vi "Nav Testing 2.0.vi"(11 "Start X":dbl) -> ()   [LabVIEW 2015]
panel:
  in  "String":string
  out "Array 5":dbl[][](array[numeric])
  out "x+y 2":dbl
  out "cornerDist1":dbl
  in  "Dest Y":dbl
  in  "Dest X":dbl
  in  "Start Y":dbl
  # "Moves robot between two specified points.\nNo localization data required.\n\nImplements basic motor control."
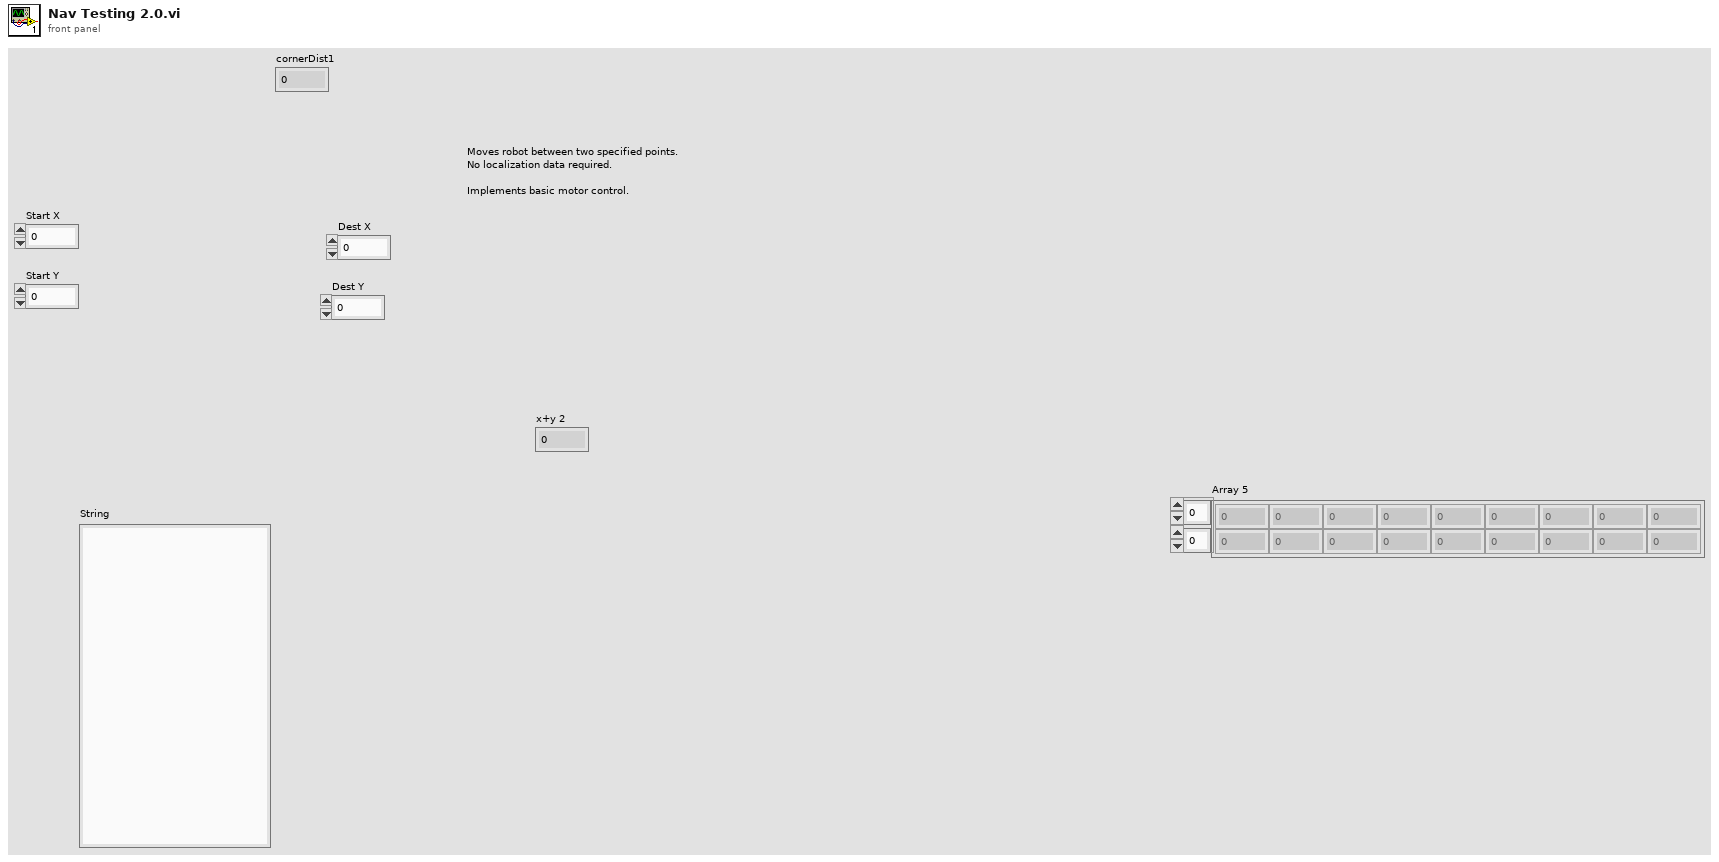
[diagram p1: front panel]
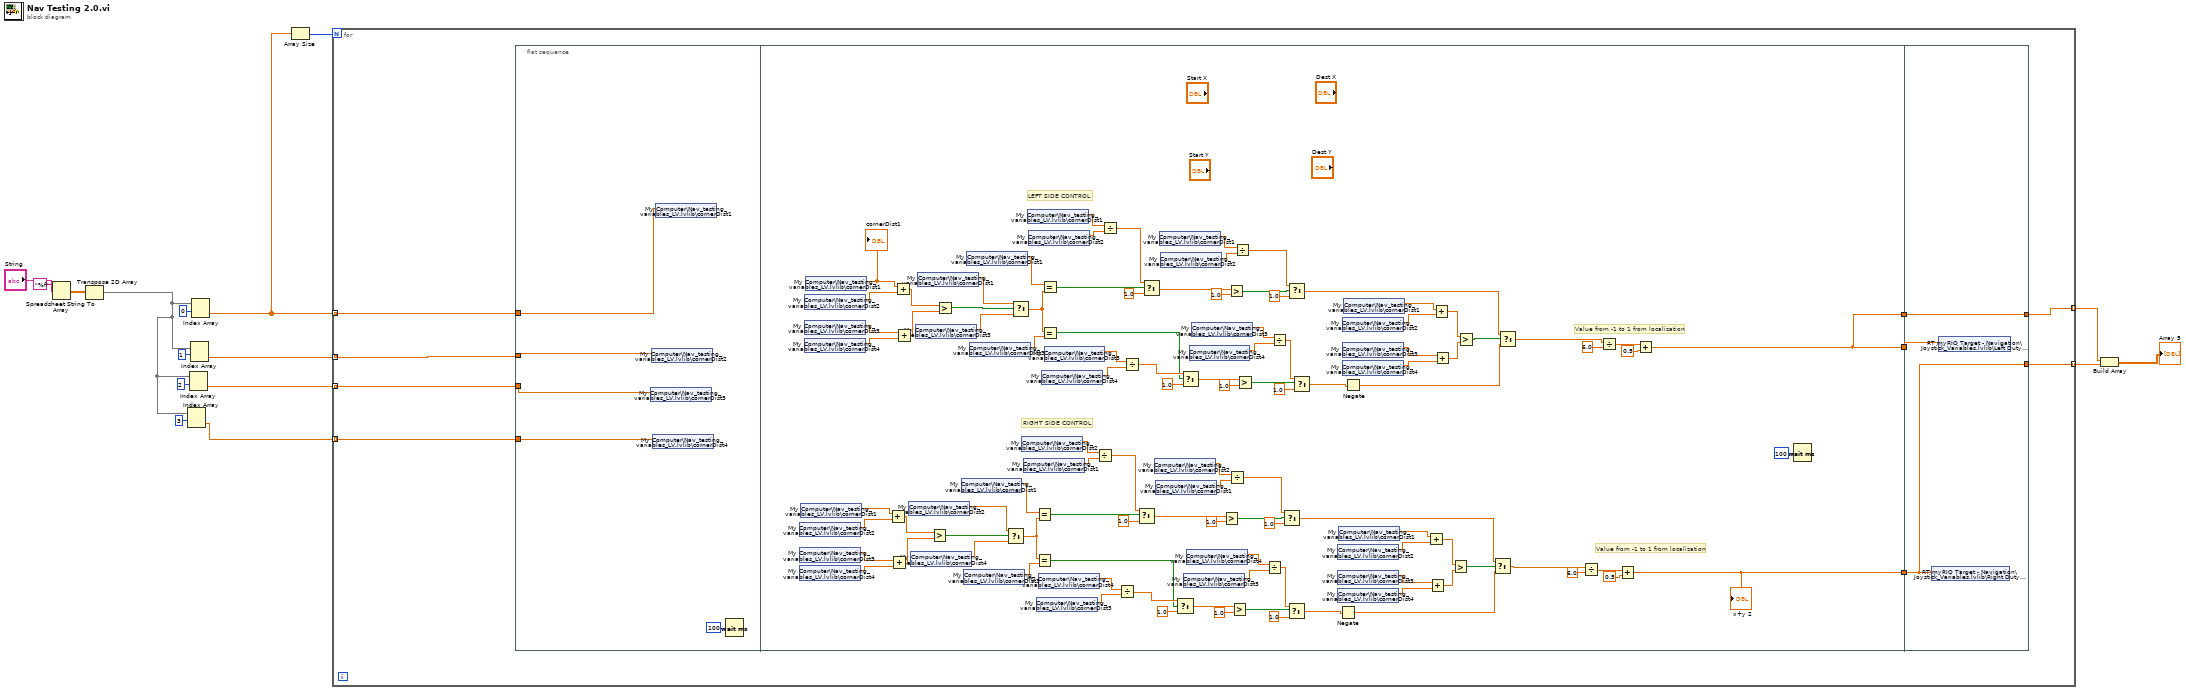
[diagram p0: block diagram]
diagram:
  n1 = Spreadsheet String To Array(format string="%f", spreadsheet string="String") -> (array=w3:dbl[][])  [unwired: 2 in]
  n2 = Transpose 2D Array(2D array=w3) -> (transposed array=w2:dbl[][])
  n3 = Index Array(array=w2, index (row)=3) -> (element=w6:dbl[])  [unwired: 1 in]
  n4 = Index Array(array=w2, index (row)=2) -> (element=w8:dbl[])  [unwired: 1 in]
  n5 = Index Array(array=w2, index (row)=1) -> (element=w10:dbl[])  [unwired: 1 in]
  n6 = Index Array(array=w2, index (row)=0) -> (element=w5:dbl[])  [unwired: 1 in]
  n7 = Array Size(array=w5) -> (size(s)=w16:i32)
  n8 = for {
    N: w16 -> [_]
    tunnel: [w22] -> w15 mode=indexing
    tunnel: w5 -> [w21] mode=indexing
    tunnel: w10 -> [w20] mode=indexing
    tunnel: w8 -> [w19] mode=indexing
    tunnel: w6 -> [w18] mode=indexing
    tunnel: [w17] -> w1 mode=indexing
    n9 = flat-sequence {
      tunnel: w21 -> [w29]
      tunnel: w20 -> [w28]
      tunnel: w19 -> [w27]
      tunnel: w18 -> [w26]
      tunnel: [w31] -> w25
      tunnel: [w32] -> w24
      tunnel: [w31] -> w23
      tunnel: w25 -> [w135]
      tunnel: w24 -> [w134]
      tunnel: w23 -> [w136]
      tunnel: [w136] -> w22
      tunnel: [w134] -> w17
      frame #0 {
        n10 = shared-variable "My Computer\\Nav_testing_variables_LV.lvlib\\cornerDist3"(w27) -> ()  [unwired: 1 in, 1 out]
        n11 = shared-variable "My Computer\\Nav_testing_variables_LV.lvlib\\cornerDist2"(w28) -> ()  [unwired: 1 in, 1 out]
        n12 = shared-variable "My Computer\\Nav_testing_variables_LV.lvlib\\cornerDist4"(w26) -> ()  [unwired: 1 in, 1 out]
        n13 = shared-variable "My Computer\\Nav_testing_variables_LV.lvlib\\cornerDist1"(w29) -> ()  [unwired: 1 in, 1 out]
        n14 = Wait (ms)(milliseconds to wait=u32 100) -> ()  [unwired: 1 out]
      }
      frame #1 {
        # "RIGHT SIDE CONTROL"
        # "LEFT SIDE CONTROL"
        # "Value from -1 to 1 from localization"
        # "Value from -1 to 1 from localization"
        n15 = shared-variable "My Computer\\Nav_testing_variables_LV.lvlib\\cornerDist2"() -> (w76:dbl)  [unwired: 1 in, 1 out]
        n16 = shared-variable "My Computer\\Nav_testing_variables_LV.lvlib\\cornerDist3"() -> (w79:dbl)  [unwired: 1 in, 1 out]
        n17 = shared-variable "My Computer\\Nav_testing_variables_LV.lvlib\\cornerDist4"() -> (w78:dbl)  [unwired: 1 in, 1 out]
        n18 = shared-variable "My Computer\\Nav_testing_variables_LV.lvlib\\cornerDist1"() -> (w77:dbl)  [unwired: 1 in, 1 out]
        n19 = shared-variable "My Computer\\Nav_testing_variables_LV.lvlib\\cornerDist2"() -> (w121:dbl)  [unwired: 1 in, 1 out]
        n20 = shared-variable "My Computer\\Nav_testing_variables_LV.lvlib\\cornerDist3"() -> (w124:dbl)  [unwired: 1 in, 1 out]
        n21 = shared-variable "My Computer\\Nav_testing_variables_LV.lvlib\\cornerDist4"() -> (w123:dbl)  [unwired: 1 in, 1 out]
        n22 = shared-variable "My Computer\\Nav_testing_variables_LV.lvlib\\cornerDist1"() -> (w122:dbl)  [unwired: 1 in, 1 out]
        "cornerDist1" <- w122
        n23 = Add(x=w77, y=w76) -> (x+y=w82:dbl)
        n24 = Add(x=w79, y=w78) -> (x+y=w81:dbl)
        n25 = Add(x=w122, y=w121) -> (x+y=w127:dbl)
        n26 = Add(x=w124, y=w123) -> (x+y=w126:dbl)
        n27 = shared-variable "My Computer\\Nav_testing_variables_LV.lvlib\\cornerDist2"() -> (w40:dbl)  [unwired: 1 in, 1 out]
        n28 = shared-variable "My Computer\\Nav_testing_variables_LV.lvlib\\cornerDist4"() -> (w75:dbl)  [unwired: 1 in, 1 out]
        n29 = shared-variable "My Computer\\Nav_testing_variables_LV.lvlib\\cornerDist3"() -> (w120:dbl)  [unwired: 1 in, 1 out]
        n30 = shared-variable "My Computer\\Nav_testing_variables_LV.lvlib\\cornerDist1"() -> (w119:dbl)  [unwired: 1 in, 1 out]
        n31 = Greater?(x=w82, y=w81) -> (0:w80:bool)
        n32 = Greater?(x=w127, y=w126) -> (0:w125:bool)
        n33 = shared-variable "My Computer\\Nav_testing_variables_LV.lvlib\\cornerDist1"() -> (w74:dbl)  [unwired: 1 in, 1 out]
        n34 = shared-variable "My Computer\\Nav_testing_variables_LV.lvlib\\cornerDist3"() -> (w72:dbl)  [unwired: 1 in, 1 out]
        n35 = shared-variable "My Computer\\Nav_testing_variables_LV.lvlib\\cornerDist1"() -> (w118:dbl)  [unwired: 1 in, 1 out]
        n36 = shared-variable "My Computer\\Nav_testing_variables_LV.lvlib\\cornerDist3"() -> (w116:dbl)  [unwired: 1 in, 1 out]
        n37 = Select(t=w40, s=w80, f=w75) -> (s? t:f=w73:dbl)
        n38 = Select(t=w119, s=w125, f=w120) -> (s? t:f=w117:dbl)
        n39 = shared-variable "My Computer\\Nav_testing_variables_LV.lvlib\\cornerDist2"() -> (w34:dbl)  [unwired: 1 in, 1 out]
        n40 = shared-variable "My Computer\\Nav_testing_variables_LV.lvlib\\cornerDist1"() -> (w71:dbl)  [unwired: 1 in, 1 out]
        n41 = shared-variable "My Computer\\Nav_testing_variables_LV.lvlib\\cornerDist1"() -> (w114:dbl)  [unwired: 1 in, 1 out]
        n42 = shared-variable "My Computer\\Nav_testing_variables_LV.lvlib\\cornerDist2"() -> (w115:dbl)  [unwired: 1 in, 1 out]
        n43 = Equal?(x=w74, y=w73) -> (x = y?=w70:bool)
        n44 = Equal?(x=w73, y=w72) -> (x = y?=w65:bool)
        n45 = shared-variable "My Computer\\Nav_testing_variables_LV.lvlib\\cornerDist3"() -> (w67:dbl)  [unwired: 1 in, 1 out]
        n46 = shared-variable "My Computer\\Nav_testing_variables_LV.lvlib\\cornerDist4"() -> (w68:dbl)  [unwired: 1 in, 1 out]
        n47 = Equal?(x=w118, y=w117) -> (x = y?=w113:bool)
        n48 = Equal?(x=w117, y=w116) -> (x = y?=w108:bool)
        n49 = shared-variable "My Computer\\Nav_testing_variables_LV.lvlib\\cornerDist4"() -> (w110:dbl)  [unwired: 1 in, 1 out]
        n50 = shared-variable "My Computer\\Nav_testing_variables_LV.lvlib\\cornerDist3"() -> (w111:dbl)  [unwired: 1 in, 1 out]
        n51 = Divide(x=w34, y=w71) -> (x/y=w69:dbl)
        n52 = Divide(x=w114, y=w115) -> (x/y=w112:dbl)
        n53 = Divide(x=w68, y=w67) -> (x/y=w66:dbl)
        n54 = Divide(x=w111, y=w110) -> (x/y=w109:dbl)
        n55 = Select(t=w69, s=w70, f=1.0) -> (s? t:f=w57:dbl)
        n56 = Select(t=w112, s=w113, f=1.0) -> (s? t:f=w100:dbl)
        n57 = shared-variable "My Computer\\Nav_testing_variables_LV.lvlib\\cornerDist2"() -> (w52:dbl)  [unwired: 1 in, 1 out]
        n58 = shared-variable "My Computer\\Nav_testing_variables_LV.lvlib\\cornerDist1"() -> (w53:dbl)  [unwired: 1 in, 1 out]
        n59 = shared-variable "My Computer\\Nav_testing_variables_LV.lvlib\\cornerDist1"() -> (w95:dbl)  [unwired: 1 in, 1 out]
        n60 = shared-variable "My Computer\\Nav_testing_variables_LV.lvlib\\cornerDist2"() -> (w96:dbl)  [unwired: 1 in, 1 out]
        n61 = Select(t=w66, s=w65, f=1.0) -> (s? t:f=w64:dbl)
        n62 = Select(t=w109, s=w108, f=1.0) -> (s? t:f=w107:dbl)
        n63 = shared-variable "My Computer\\Nav_testing_variables_LV.lvlib\\cornerDist3"() -> (w61:dbl)  [unwired: 1 in, 1 out]
        n64 = shared-variable "My Computer\\Nav_testing_variables_LV.lvlib\\cornerDist4"() -> (w62:dbl)  [unwired: 1 in, 1 out]
        n65 = shared-variable "My Computer\\Nav_testing_variables_LV.lvlib\\cornerDist4"() -> (w104:dbl)  [unwired: 1 in, 1 out]
        n66 = shared-variable "My Computer\\Nav_testing_variables_LV.lvlib\\cornerDist3"() -> (w105:dbl)  [unwired: 1 in, 1 out]
        n67 = Greater?(x=w57, y=1.0) -> (0:w55:bool)
        n68 = Greater?(x=w100, y=1.0) -> (0:w98:bool)
        n69 = Divide(x=w52, y=w53) -> (x/y=w51:dbl)
        n70 = Greater?(x=w64, y=1.0) -> (0:w60:bool)
        n71 = Divide(x=w95, y=w96) -> (x/y=w94:dbl)
        n72 = Greater?(x=w107, y=1.0) -> (0:w103:bool)
        n73 = Divide(x=w62, y=w61) -> (x/y=w59:dbl)
        n74 = Divide(x=w105, y=w104) -> (x/y=w102:dbl)
        n75 = Select(t=w51, s=w55, f=1.0) -> (s? t:f=w44:dbl)
        n76 = Select(t=w59, s=w60, f=1.0) -> (s? t:f=w42:dbl)
        n77 = Select(t=w94, s=w98, f=1.0) -> (s? t:f=w87:dbl)
        n78 = Select(t=w102, s=w103, f=1.0) -> (s? t:f=w84:dbl)
        n79 = shared-variable "My Computer\\Nav_testing_variables_LV.lvlib\\cornerDist2"() -> (w47:dbl)  [unwired: 1 in, 1 out]
        n80 = shared-variable "My Computer\\Nav_testing_variables_LV.lvlib\\cornerDist3"() -> (w50:dbl)  [unwired: 1 in, 1 out]
        n81 = shared-variable "My Computer\\Nav_testing_variables_LV.lvlib\\cornerDist4"() -> (w49:dbl)  [unwired: 1 in, 1 out]
        n82 = shared-variable "My Computer\\Nav_testing_variables_LV.lvlib\\cornerDist1"() -> (w48:dbl)  [unwired: 1 in, 1 out]
        n83 = Negate(x=w42) -> (-x=w41:dbl)
        n84 = shared-variable "My Computer\\Nav_testing_variables_LV.lvlib\\cornerDist2"() -> (w90:dbl)  [unwired: 1 in, 1 out]
        n85 = shared-variable "My Computer\\Nav_testing_variables_LV.lvlib\\cornerDist3"() -> (w93:dbl)  [unwired: 1 in, 1 out]
        n86 = shared-variable "My Computer\\Nav_testing_variables_LV.lvlib\\cornerDist4"() -> (w92:dbl)  [unwired: 1 in, 1 out]
        n87 = shared-variable "My Computer\\Nav_testing_variables_LV.lvlib\\cornerDist1"() -> (w91:dbl)  [unwired: 1 in, 1 out]
        n88 = Negate(x=w84) -> (-x=w83:dbl)
        n89 = Add(x=w48, y=w47) -> (x+y=w46:dbl)
        n90 = Add(x=w50, y=w49) -> (x+y=w45:dbl)
        n91 = Add(x=w91, y=w90) -> (x+y=w89:dbl)
        n92 = Add(x=w93, y=w92) -> (x+y=w88:dbl)
        n93 = Greater?(x=w46, y=w45) -> (0:w43:bool)
        n94 = Greater?(x=w89, y=w88) -> (0:w86:bool)
        n95 = Select(t=w44, s=w43, f=w41) -> (s? t:f=w39:dbl)
        n96 = Select(t=w87, s=w86, f=w83) -> (s? t:f=w85:dbl)
        n97 = Divide(x=w39, y=6.0) -> (x/y=w132:dbl)
        n98 = Divide(x=w85, y=6.0) -> (x/y=w129:dbl)
        n99 = Add(x=w132, y=0.5) -> (x+y=w32:dbl)
        "x+y 2" <- w32
        n100 = Add(x=w129, y=0.5) -> (x+y=w31:dbl)
        n101 = Wait (ms)(milliseconds to wait=u32 100) -> ()  [unwired: 1 out]
      }
      frame #2 {
        n102 = shared-variable "RT myRIO Target - Navigation\\Joystick_Variables.lvlib\\Right Duty Cycle"(w134) -> ()  [unwired: 1 in, 1 out]
        n103 = shared-variable "RT myRIO Target - Navigation\\Joystick_Variables.lvlib\\Left Duty Cycle"(w135) -> ()  [unwired: 1 in, 1 out]
      }
    }
  }
  n104 = Build Array(w15, w1) -> (→"Array 5":dbl[][])
